vi "MakeRoom.vi"(8 "error in (no error)":errorcluster, 10 "RoomNumber":i32, 11 "EnchantedMazeGame":refnum<class "EnchantedMazeGame.lvclass">) -> (0 "error out":errorcluster, 2 "Room":refnum<class "Room.lvclass">, 3 "EnchantedMazeGame":refnum<class "EnchantedMazeGame.lvclass">)   [LabVIEW 2020, in "FactoryMethod.lvlib" / "NoParametrizedFactoryMethod.lvlib" / "EnchantedMazeGame.lvclass"]
uses:
  EnchantedMazeGame.lvclass
  GoFcommonClasses/ConcreteMazeSite/Room/Room.lvclass
  GoFcommonClasses/ConcreteMazeSite/EnchantedRoom/EnchantedRoom.lvclass
  E:/Francesco/GitHub/Design-Patterns-GoF_-_NI-LV/Creational/GoFcommonClasses/ConcreteMazeSite/Room/Room.lvclass
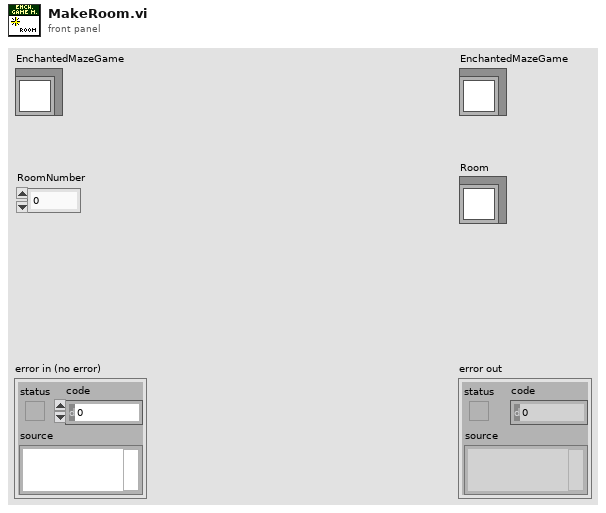
[diagram p1: front panel]
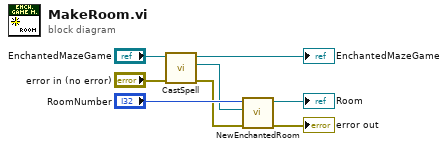
[diagram p0: block diagram]
diagram:
  n1 = call "CastSpell.vi"("error in (no error)"="error in (no error)", "EnchantedMazeGame in"="EnchantedMazeGame") -> ("error out"=w1:errorcluster, "Spell"=w3:refnum<class "Spell.lvclass">, "EnchantedMazeGame out"=→"EnchantedMazeGame":refnum<class "EnchantedMazeGame.lvclass">)  [unwired: 7 in]
  n2 = call "NewEnchantedRoom.vi"("error in (no error)"=w1, "Spell"=w3, "RoomNumber"="RoomNumber") -> ("error out"=→"error out":errorcluster, "EnchantedRoom"=→"Room":refnum<class "EnchantedRoom.lvclass">)  [unwired: 7 in]
